vi "run.vi"(8 "error in (no error)":errorcluster, 11 "ScanModeTS090821Circular2D in":refnum<class "ImagingModeTS090821Circular2D.lvclass">) -> (0 "error out":errorcluster, 3 "ScanModeTS090821Circular2D out":refnum<class "ImagingModeTS090821Circular2D.lvclass">)   [LabVIEW 2010, in "ImagingModeTS090821Circular2D.lvclass"]
uses:
  ImagingModeTS090821Circular2D.lvclass
  common/classes/Image/Image/Image.lvclass
  GenericImagingMode/GenericImagingMode/GenericImagingMode.lvclass
  ImagingModeDL091001Scaffold/ImagingModeDL091001Scaffold/ImagingModeDL091001Scaffold.lvclass
  ImagingModeDL091001Scaffold/ImagingModeDL091001Scaffold_statechart.lvsc/Trigger.ctl
  ImagingModeDL091001Scaffold/ImagingModeDL091001Scaffold_statechart.lvsc
  bricks/enumerations/control_status.ctl
panel:
  in  "Tab Control":enum32{"User", "Debug", "About"}(tab)
  in  "save settings button":bool
  in  "load settings button":bool
  in  "number of cycles":i32=100
  in  "default settings":string(combo)
  in  "load image button":bool
  out "reference image":T1(plugin-control)
  in  "y amplitude":dbl[unit]=9.999999999999999e-06
  in  "x frequency":dbl=1.0
  in  "y frequency":dbl=1.0
  in  "phase shift":dbl
  in  "number of pixels per cycle":i32=250 min=0
  in  "x amplitude":dbl[unit]=9.999999999999999e-06
  in  "y center":dbl
  in  "x center":dbl
  in  "z center":dbl
  in  "rotation angle":dbl
  in  "type of trajectory":T2(radio)=enum."line (2-click)"
  in  "lines / frame":i32
  in  "spiral?":bool
  in  "dump factor":dbl=1.1
  in  "scanning frequency":dbl[unit]=5.0 min=0.0
  in  "pixel dwell time":dbl[unit]
  out "current frame":i32
  in  "Double":bool
  out "event loop error":errorcluster
  out "event handling loop counter":i32=10
  out "Type":i32(ring) items=["No Event"=0, "Click Event"=1, "Draw Event"=2, "Size Event"=4, "Scroll Event"=5, "Double Click Event"=8]
  out "Coordinates":i32[](array[numeric])
  in  "status":T3
  out "Tool":i32(ring) items=["None", "Selection Tool", "Point Tool", "Line Tool", "Rectangle Tool", "Oval Tool", "Polygon Tool", "ClosedFreehandTool", "Annulus Tool", "Rotated Rectangle Tool", "Zoom Tool", "Pan Tool", "Polyline Tool", "Freehand Tool"]
  out "finished?":bool
  out "x = y?":bool
  # "trajectory parameters"
  # "scan parameters"
  # "centering"
  # "spiral"
  # "ImagingModeTS090821Circular2D"
  # "Implemented by:\nTomasz Soltysinski, University Hospital Zurich, Switzerland"
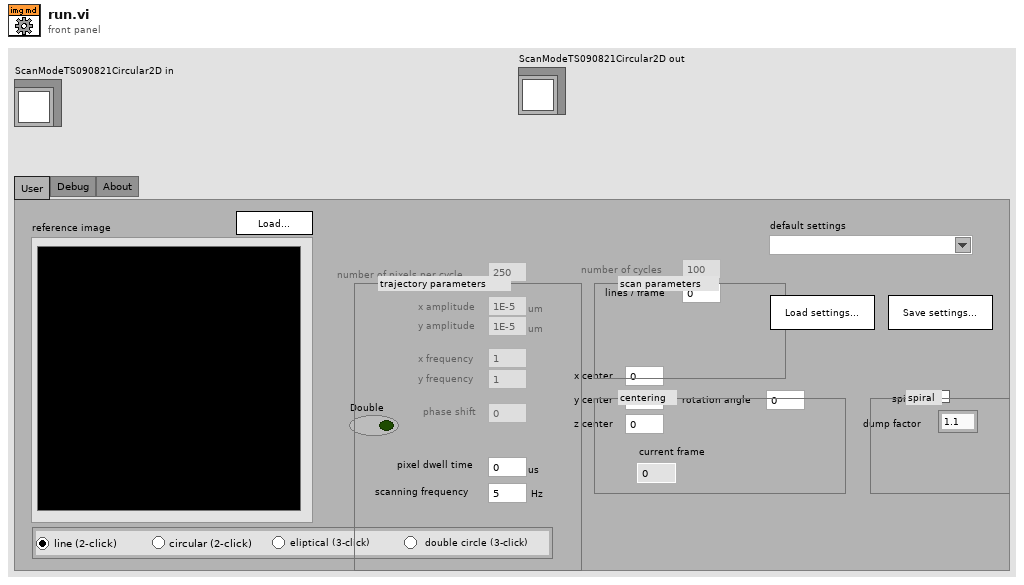
[diagram p1: front panel]
types:
  T1 = typedef "IMAQ Image.ctl" = refnum<image>
  T2 = enum32{"No Selection", "line (2-click)", "circular (2-click)", "eliptical (3-click)", "double circle (3-click)"}
  T3 = typedef "control_status.ctl" = enum16{"enabled", "disabled", "disabled & greyed out"}
  T4 = typedef "ImagingModeDL091001Scaffold_statechart.lvsc/Trigger.ctl" = enum16{"NULL", "initialise", "terminate", "start sweep", "stop sweep", "update", "proceed", "draw overlay"}
  T5 = enum8{"Enabled", "Disabled", "Disabled and Grayed Out"}
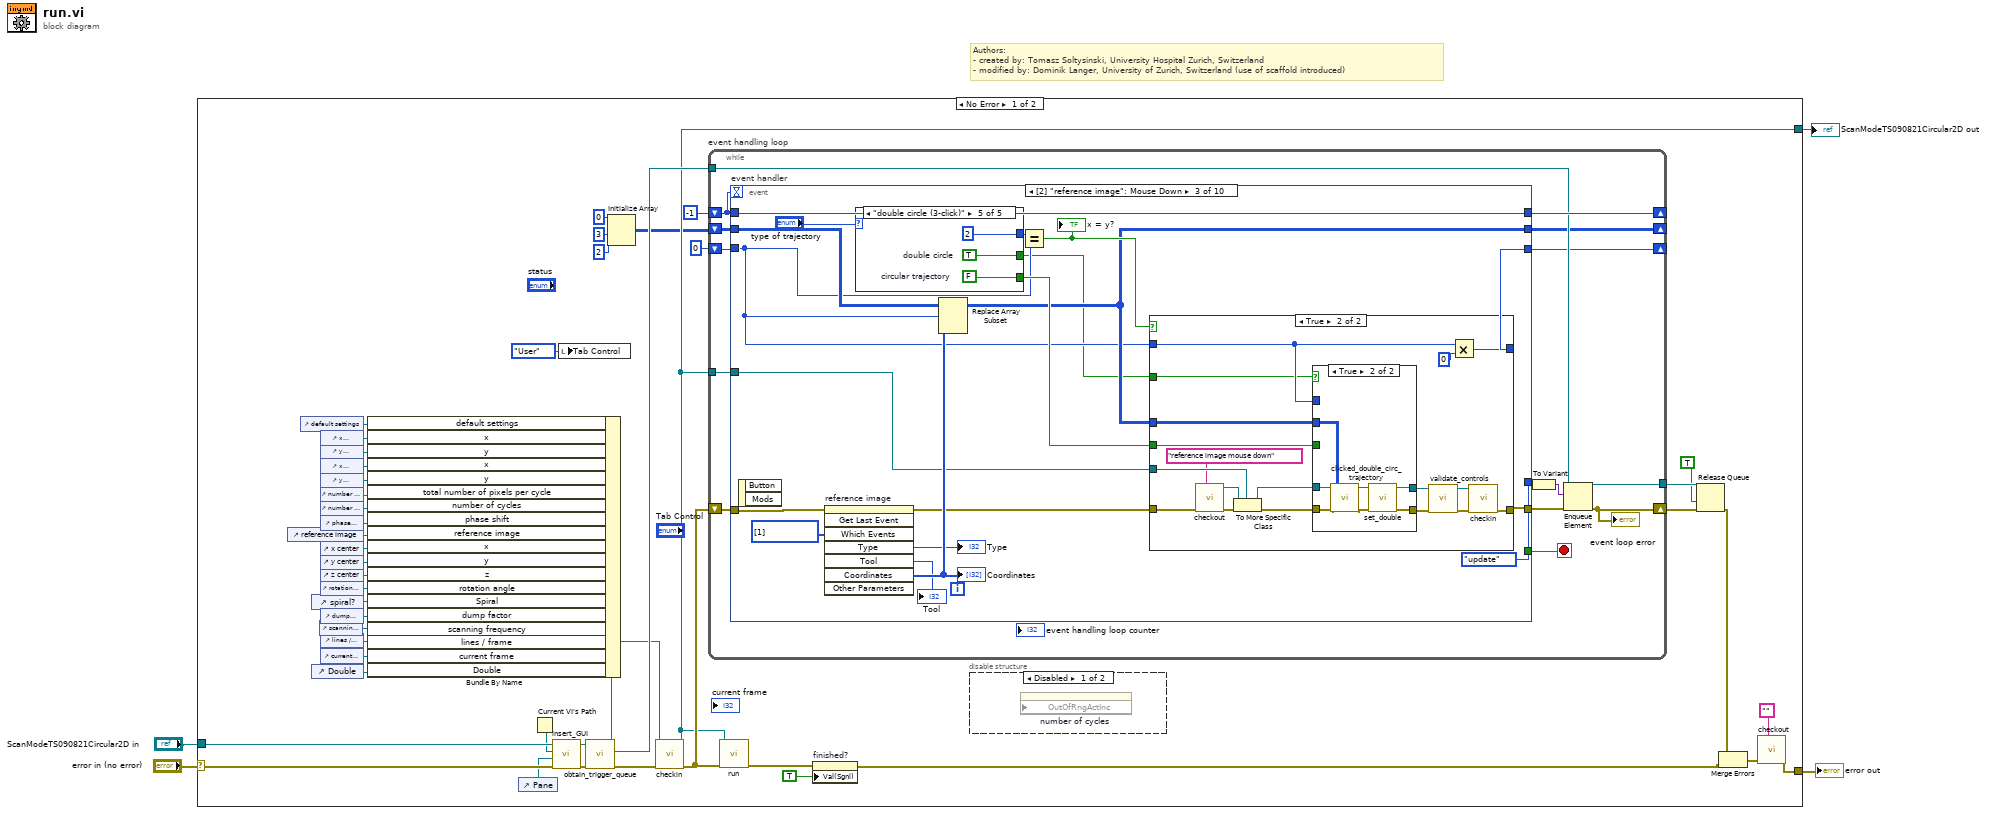
[diagram p0: block diagram]
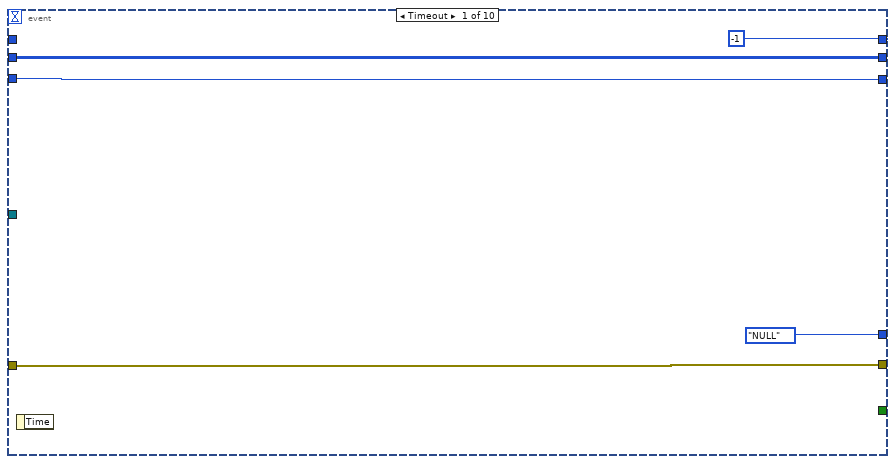
[diagram p3: hidden frame]
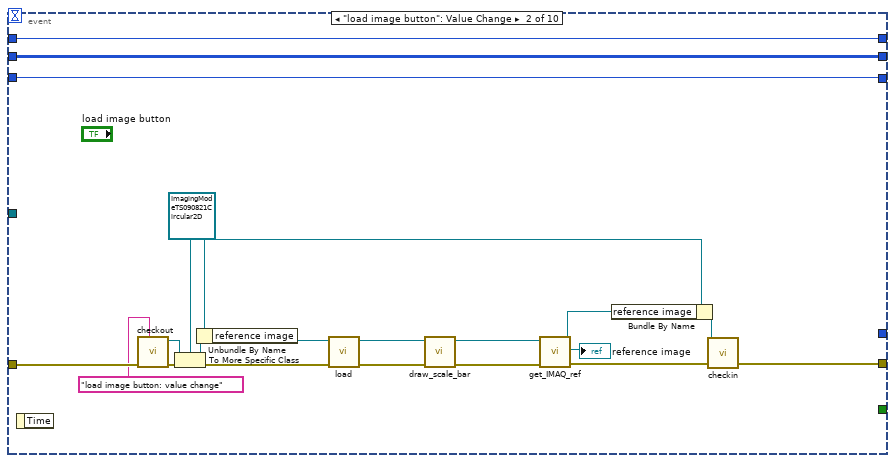
[diagram p4: hidden frame]
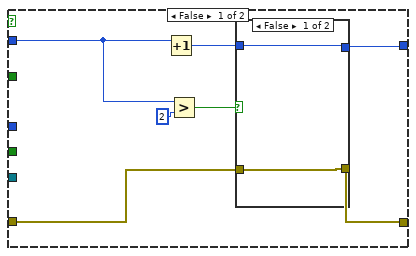
[diagram p5: hidden frame]
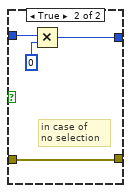
[diagram p6: hidden frame]
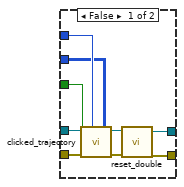
[diagram p7: hidden frame]
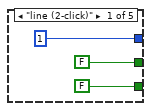
[diagram p8: hidden frame]
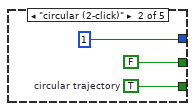
[diagram p9: hidden frame]
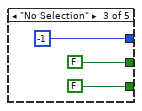
[diagram p10: hidden frame]
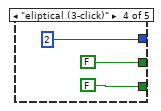
[diagram p11: hidden frame]
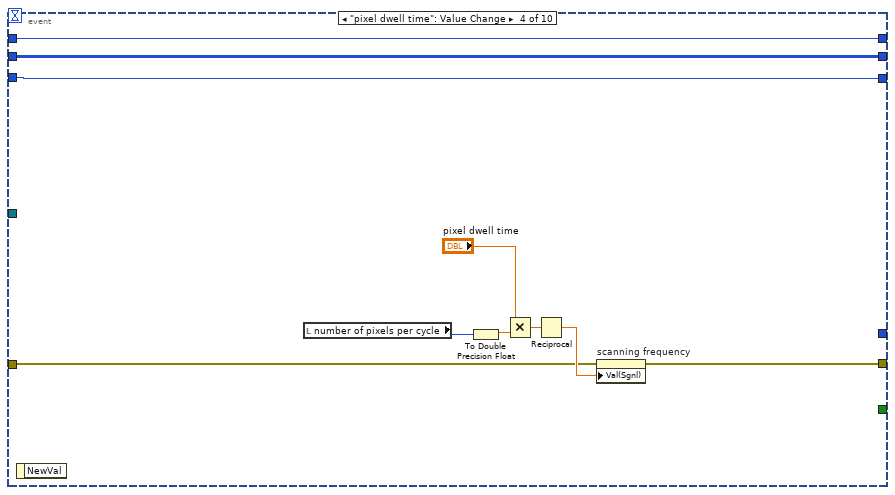
[diagram p12: hidden frame]
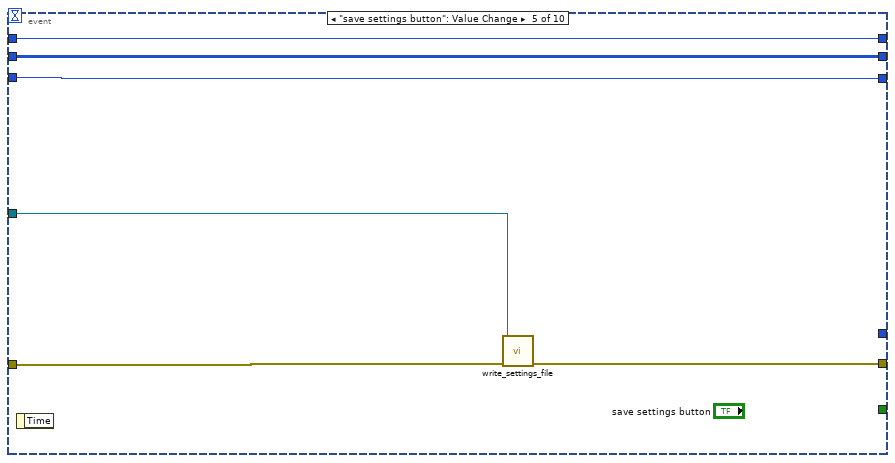
[diagram p13: hidden frame]
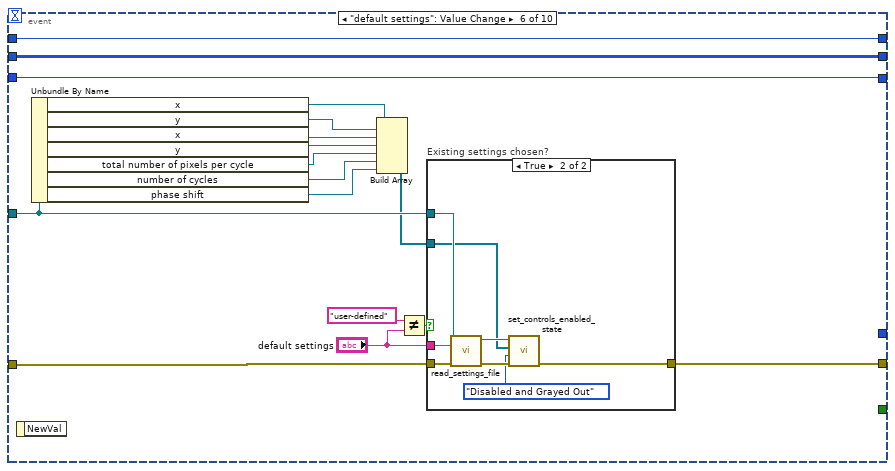
[diagram p14: hidden frame]
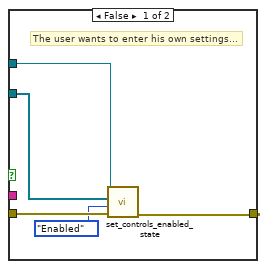
[diagram p15: hidden frame]
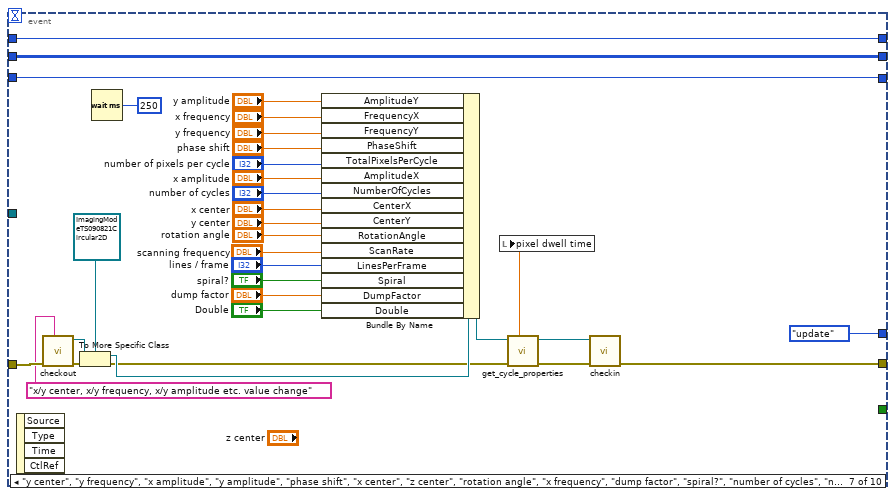
[diagram p16: hidden frame]
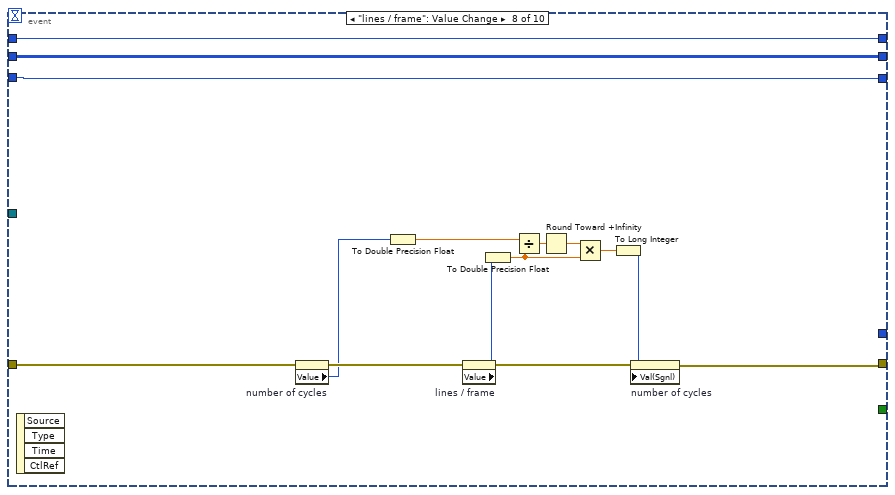
[diagram p17: hidden frame]
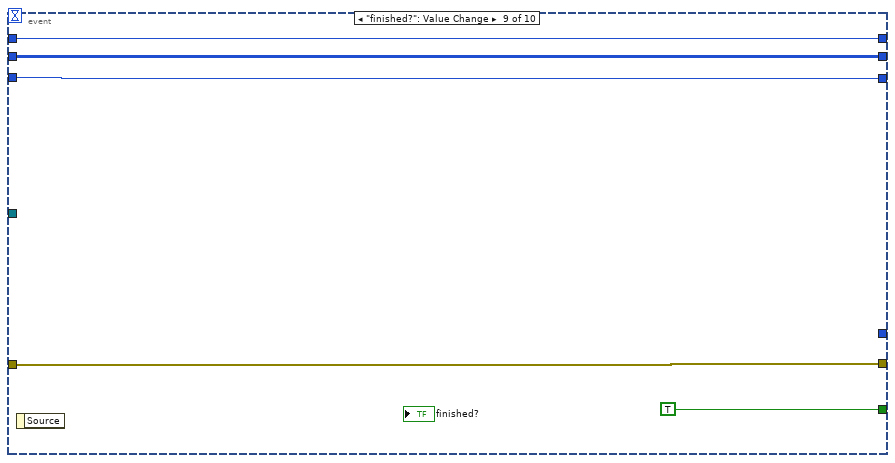
[diagram p18: hidden frame]
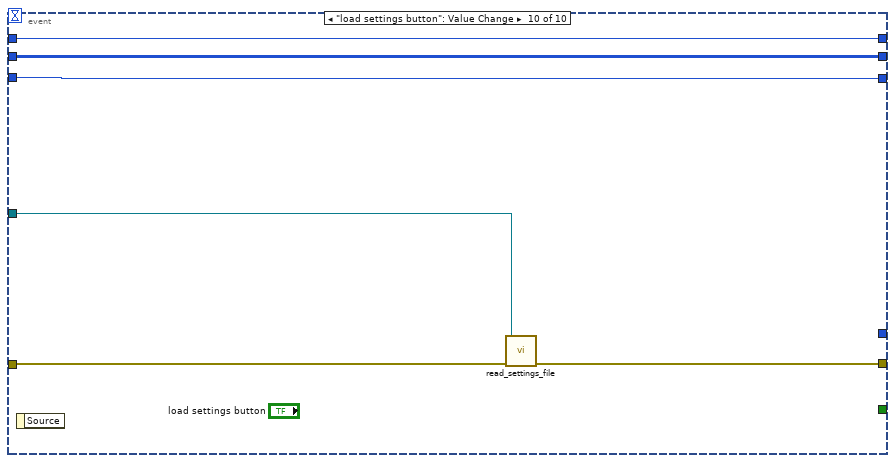
[diagram p19: hidden frame]
diagram:
  # "Authors: \n- created by: Tomasz Soltysinski, University Hospital Zurich, Switzerland\n- modified by: Dominik Langer, University of Zurich, Switzerland (use of scaffold introduced)"
  n1 = case shown="No Error" "error in (no error)" {
    selector: "error in (no error)" -> [w10 w279]
    tunnel: [w14 w279] -> w4
    tunnel: [w40 w278] -> w1
    tunnel: "ScanModeTS090821Circular2D in" -> [w9 w278]
    frame No Error {
      n2 = control-ref of="reference image"() -> (w26:refnum<vi>)
      n3 = control-ref of="default settings"() -> (w28:refnum<vi>)
      n4 = control-ref of="spiral?"() -> (w25:refnum<vi>)
      n5 = control-ref of="Double"() -> (w7:refnum<vi>)
      n6 = control-ref of="scanning frequency"() -> (w20:refnum<vi>)
      n7 = control-ref of="x amplitude"() -> (w35:refnum<vi>)
      n8 = control-ref of="y amplitude"() -> (w34:refnum<vi>)
      n9 = control-ref of="x frequency"() -> (w33:refnum<vi>)
      n10 = control-ref of="y frequency"() -> (w32:refnum<vi>)
      n11 = control-ref of="number of pixels per cycle"() -> (w31:refnum<vi>)
      n12 = control-ref of="number of cycles"() -> (w30:refnum<vi>)
      n13 = control-ref of="phase shift"() -> (w29:refnum<vi>)
      n14 = control-ref of="x center"() -> (w24:refnum<vi>)
      n15 = control-ref of="y center"() -> (w23:refnum<vi>)
      n16 = control-ref of="z center"() -> (w22:refnum<vi>)
      n17 = control-ref of="rotation angle"() -> (w27:refnum<vi>)
      n18 = control-ref of="dump factor"() -> (w21:refnum<vi>)
      n19 = control-ref of="lines / frame"() -> (w19:refnum<vi>)
      n20 = control-ref of="current frame"() -> (w18:refnum<vi>)
      n21 = control-ref of="Pane"() -> (w5:refnum<vi>)
      n22 = Current VI's Path() -> (path=w8:path)
      n23 = call-dynamic "insert_GUI.vi"("error in (no error)"=w10, "Pane"=w5, "VI path"=w8, "GenericComponent in"=w9) -> ("error out"=w12:errorcluster, "GenericComponent out"=w11:refnum<class "ImagingModeTS090821Circular2D.lvclass">)  [unwired: 6 in]
      n24 = local write "Tab Control"(enum32{"User", "Debug", "About"}."User" ("Tab Control")) -> ()
      n25 = call-dynamic "obtain_trigger_queue.vi"("error in (no error)"=w12, "GenericPlugin in"=w11) -> ("error out"=w43:errorcluster, "trigger queue"=w41:refnum<queue>, "GenericPlugin out"=w17:refnum<class "ImagingModeTS090821Circular2D.lvclass">)  [unwired: 7 in]
      n26 = Bundle By Name(cluster=w17, "default settings"=w28, "x"=w35, "y"=w34, "x"=w33, "y"=w32, "total number of pixels per cycle"=w31, "number of cycles"=w30, "phase shift"=w29, "reference image"=w26, "x"=w24, "y"=w23, "z"=w22, "rotation angle"=w27, "Spiral"=w25, "dump factor"=w21, "scanning frequency"=w20, "lines / frame"=w19, "current frame"=w18, "Double"=w7) -> (w16:refnum<class "ImagingModeTS090821Circular2D.lvclass">)
      n27 = Initialize Array(0, 3 ("dimension size"), 2 ("dimension size")) -> (w36:i32[][])
      n28 = call "checkin.vi"("error in (no error)"=w43, "GenericScanMode in"=w16) -> ("error out"=w42:errorcluster, "GenericScanMode out"=w40:refnum<class "ImagingModeTS090821Circular2D.lvclass">)  [unwired: 8 in]
      n29 = while "event handling loop" {
        shift-right: [w66] -> _
        shift-left: -1 -> [w67]
        shift-right: [w59] -> w51
        shift-left: w42 -> [w65]
        tunnel: w41 -> [w63]
        tunnel: [w61] -> w50
        tunnel: w40 -> [w60]
        shift-right: [w58] -> _
        shift-left: w36 -> [w57]
        shift-right: [w55] -> _
        shift-left: 0 -> [w56]
        stop <- w64 stop-if-true
        n30 = event "event handler" shown="[2] \"reference image\": Mouse Down" {
          selector: _ -> [_ _ _ _ _ _ _ _ _ _]
          dyn-events: _ -> [_ _ _ _ _ _ _ _ _ _]
          timeout: w67 -> [_ _ _ _ _ _ _ _ _ _]
          tunnel: [-1 w92 w111 w183 w189 w206 w251 w266 w271 w277] -> w66
          tunnel: w67 -> [_ w92 w111 w183 w189 w206 w251 w266 w271 w277]
          tunnel: w65 -> [w71 w87 w103 w176 w188 w205 w239 w262 w270 w275]
          tunnel: [w71 w79 w106 w180 w187 w204 w238 w252 w270 w274] -> w62
          tunnel: [_ _ _ _ _ _ _ _ TRUE _] -> w64
          tunnel: w60 -> [_ _ w96 _ w186 w191 _ _ _ w276]
          tunnel: [Trigger."NULL" ("Trigger") _ Trigger."update" ("Trigger") _ _ _ Trigger."update" ("Trigger") _ _ _] -> w54
          tunnel: [w70 w81 w107 w182 w185 w200 w234 w265 w268 w273] -> w58
          tunnel: w57 -> [w70 w81 w102 w182 w185 w200 w234 w265 w268 w273]
          tunnel: w56 -> [w69 w80 w100 w181 w184 w199 w233 w264 w267 w272]
          tunnel: [w69 w80 w104 w181 w184 w199 w233 w264 w267 w272] -> w55
          event Timeout {
            n31 = event-data() -> ()  [unwired: 2 out]
          }
          event "load image button": Value Change {
            n32 = event-data() -> ()  [unwired: 2 out]
            n33 = call "checkout.vi"("locked by?"="load image button: value change", "error in (no error)"=w87) -> ("error out"=w91:errorcluster, "GenericScanMode out"=w90:refnum<class "GenericImagingMode.lvclass">)  [unwired: 8 in]
            n34 = To More Specific Class(target class=refnum<class "ImagingModeTS090821Circular2D.lvclass"> refnum ("ScanModeTS090821Circular2D.lvclass"), reference=w90, error in=w91) -> (specific class reference=w82:refnum<class "ImagingModeTS090821Circular2D.lvclass">, error out=w86:errorcluster)
            n35 = Unbundle By Name(w82) -> ("reference image"=w88:refnum<class "Image.lvclass">)
            n36 = call-dynamic "load.vi"("error in (no error)"=w86, "Image in"=w88) -> ("error out"=w76:errorcluster, "Image out"=w74:refnum<class "Image.lvclass">)  [unwired: 6 in, 2 out]
            n37 = call "draw_scale_bar.vi"("error in (no error)"=w76, "Image in"=w74) -> ("error out"=w75:errorcluster, "Image out"=w73:refnum<class "Image.lvclass">)  [unwired: 8 in]
            n38 = call-dynamic "get_IMAQ_ref.vi"("error in (no error)"=w75, "Image.lvclass in"=w73) -> ("error out"=w78:errorcluster, "Image"=→"reference image":T1, "Image.lvclass out"=w85:refnum<class "Image.lvclass">)  [unwired: 5 in, 2 out]
            n39 = Bundle By Name(cluster=w82, "reference image"=w85) -> (w77:refnum<class "ImagingModeTS090821Circular2D.lvclass">)
            n40 = call "checkin.vi"("error in (no error)"=w78, "GenericScanMode in"=w77) -> ("error out"=w79:errorcluster)  [unwired: 8 in, 1 out]
          }
          event "reference image": Mouse Down {
            w97 = i32[] [1] items=["No  event", "Click event", "Draw event", "Move event", "Size event", "Scroll event", "Activate event", "Close event", "Double click event"] ("Events list (all)")
            n41 = event-data() -> ()  [unwired: 3 out]
            n42 = invoke on="reference image" class="ImageControl" method="Get Last Event"(error in=w103, "Which Events"=w97) -> (error out=w95:errorcluster, "Type"=→"Type":i32, "Tool"=→"Tool":i32, "Coordinates"=w101:i32[])  [unwired: 6 in, 4 out]
            "Coordinates" <- w101
            n43 = case shown="\"double circle (3-click)\"" "type of trajectory" {
              tunnel: [1 1 -1 2 2] -> w110
              tunnel: [FALSE w163 FALSE ("circular trajectory") FALSE ("circular trajectory") w172] -> w109
              tunnel: [FALSE ("double circle") FALSE ("double circle") FALSE ("double circle") FALSE ("double circle") w171] -> w94
              frame "line (2-click)" {
              }
              frame "circular (2-click)" {
                w163 = TRUE  # circular trajectory
              }
              frame "No Selection" {
              }
              frame "eliptical (3-click)" {
              }
              frame "double circle (3-click)" {
                w171 = TRUE  # double circle
                w172 = FALSE  # circular trajectory
              }
            }
            n44 = Replace Array Subset(array=w102, new element=w101, index (row)=w100) -> (w107:i32[][])  [unwired: 1 in]
            n45 = Equal?(x=w110, y=w100) -> (x = y?=w108:bool)
            "x = y?" <- w108
            n46 = case shown="True" w108 {
              tunnel: [w117 w142] -> w104
              tunnel: w100 -> [w113 w140]
              tunnel: w107 -> [_ w139]
              tunnel: w96 -> [_ w131]
              tunnel: w95 -> [w115 w135]
              tunnel: [w114 w129] -> w106
              tunnel: w109 -> [_ w138]
              tunnel: w94 -> [_ w125]
              frame False {
                n47 = Increment(x=w113) -> (x+1=w118:i32)
                n48 = Greater?(x=w113, y=2) -> (0:w116:bool)
                n49 = case shown="False" w116 {
                  tunnel: w118 -> [w120 w123]
                  tunnel: [w120 w122] -> w117
                  tunnel: w115 -> [w119 w121]
                  tunnel: [w119 w121] -> w114
                  frame False {
                  }
                  frame True {
                    # "in case of\nno selection"
                    n50 = Multiply(x=w123, y=0 ("x")) -> (x*y=w122:i32)
                  }
                }
              }
              frame True {
                n51 = call "checkout.vi"("locked by?"="reference image mouse down", "error in (no error)"=w135) -> ("error out"=w134:errorcluster, "GenericScanMode out"=w132:refnum<class "GenericImagingMode.lvclass">)  [unwired: 8 in]
                n52 = To More Specific Class(target class=w131, reference=w132, error in=w134) -> (specific class reference=w127:refnum<class "ImagingModeTS090821Circular2D.lvclass">, error out=w133:errorcluster)
                n53 = case shown="True" w125 {
                  tunnel: w140 -> [w151 _]
                  tunnel: w139 -> [w150 w157]
                  tunnel: w138 -> [w149 _]
                  tunnel: [w143 w154] -> w137
                  tunnel: [w145 w152] -> w136
                  tunnel: w133 -> [w148 w158]
                  tunnel: w127 -> [w147 w156]
                  frame False {
                    n54 = call-dynamic "clicked_trajectory.vi"("ScanModeTS090821Circular2D in"=w147, "clicked points"=w150, "Numeric"=w151, "circular trajectory"=w149, "error in (no error)"=w148) -> ("ScanModeTS090821Circular2D out"=w146:refnum<class "ImagingModeTS090821Circular2D.lvclass">, "error out"=w144:errorcluster)  [unwired: 21 in]
                    n55 = call-dynamic "reset_double.vi"("error in (no error)"=w144, "ImagingModeTS090821Circular2D in"=w146) -> ("error out"=w143:errorcluster, "ImagingModeTS090821Circular2D out"=w145:refnum<class "ImagingModeTS090821Circular2D.lvclass">)  [unwired: 8 in]
                  }
                  frame True {
                    n56 = call-dynamic "clicked_double_circ_trajectory.vi"("ScanModeTS090821Circular2D in"=w156, "clicked points"=w157, "error in (no error)"=w158) -> ("ScanModeTS090821Circular2D out"=w153:refnum<class "ImagingModeTS090821Circular2D.lvclass">, "error out"=w155:errorcluster)  [unwired: 23 in]
                    n57 = call-dynamic "set_double.vi"("error in (no error)"=w155, "ImagingModeTS090821Circular2D in"=w153) -> ("error out"=w154:errorcluster, "ImagingModeTS090821Circular2D out"=w152:refnum<class "ImagingModeTS090821Circular2D.lvclass">)  [unwired: 8 in]
                  }
                }
                n58 = call-dynamic "validate_controls.vi"("error in (no error)"=w137, "ScanModeTS090821Circular2D in"=w136) -> ("error out"=w130:errorcluster, "ScanModeTS090821Circular2D out"=w128:refnum<class "ImagingModeTS090821Circular2D.lvclass">)  [unwired: 8 in]
                n59 = Multiply(x=w140, y=0) -> (x*y=w142:i32)
                n60 = call "checkin.vi"("error in (no error)"=w130, "GenericScanMode in"=w128) -> ("error out"=w129:errorcluster)  [unwired: 8 in, 1 out]
              }
            }
          }
          event "pixel dwell time": Value Change {
            n61 = event-data() -> ()  [unwired: 2 out]
            n62 = local read "number of pixels per cycle"() -> (w175:i32)
            n63 = To Double Precision Float(number=w175) -> (double precision float=w179:dbl)
            n64 = Multiply(x="pixel dwell time", y=w179) -> (x*y=w178:dbl[unit])
            n65 = Reciprocal(x=w178) -> (1/x=w177:dbl[unit])
            n66 = property on="scanning frequency" class="DigNum (strict)"(error in=w176, "Val(Sgnl)"=w177) -> (error out=w180:errorcluster)  [unwired: 1 in, 1 out]
          }
          event "save settings button": Value Change {
            n67 = event-data() -> ()  [unwired: 2 out]
            n68 = call-dynamic "write_settings_file.vi"("error in (no error)"=w188, "GenericPlugin in"=w186) -> ("error out"=w187:errorcluster)  [unwired: 6 in, 3 out]
          }
          event "default settings": Value Change {
            n69 = event-data() -> ()  [unwired: 2 out]
            n70 = Unbundle By Name(w191) -> ("x"=w198:refnum<vi>, "y"=w197:refnum<vi>, "x"=w196:refnum<vi>, "y"=w195:refnum<vi>, "total number of pixels per cycle"=w194:refnum<vi>, "number of cycles"=w193:refnum<vi>, "phase shift"=w192:refnum<vi>)
            n71 = Build Array(w198, w197, w196, w195, w194, w193, w192) -> (w190:refnum<vi>[])
            n72 = Not Equal?(x="user-defined", y="default settings") -> (x != y?=w202:bool)
            n73 = case "Existing settings chosen?" shown="True" w202 {
              tunnel: w191 -> [w210 w215]
              tunnel: w205 -> [w211 w217]
              tunnel: [w209 w219] -> w204
              tunnel: "default settings" -> [_ w214]
              tunnel: w190 -> [w207 w212]
              frame False {
                # "The user wants to enter his own settings..."
                n74 = call-dynamic "set_controls_enabled_state.vi"("error in (no error)"=w211, "status"=T5."Enabled", "control references"=w207, "GenericPlugin in"=w210) -> ("error out"=w209:errorcluster)  [unwired: 6 in, 1 out]
              }
              frame True {
                n75 = call-dynamic "read_settings_file.vi"("error in (no error)"=w217, "settings name"=w214, "ScanModeTS090821Circular2D in"=w215) -> ("error out"=w218:errorcluster, "ScanModeTS090821Circular2D out"=w216:refnum<class "ImagingModeTS090821Circular2D.lvclass">)  [unwired: 6 in, 1 out]
                n76 = call-dynamic "set_controls_enabled_state.vi"("error in (no error)"=w218, "status"=T5."Disabled and Grayed Out", "control references"=w212, "GenericPlugin in"=w216) -> ("error out"=w219:errorcluster)  [unwired: 6 in, 1 out]
              }
            }
          }
          event "y center", "y frequency", "x amplitude", "y amplitude", "phase shift", "x center", "z center", "rotation angle", "x frequency", "dump factor", "spiral?", "number of cycles", "number of pixels per cycle", "scanning frequency": Value Change {
            n77 = event-data() -> ()  [unwired: 5 out]
            n78 = call "checkout.vi"("locked by?"="x/y center, x/y frequency, x/y amplitude etc. value change", "error in (no error)"=w239) -> ("error out"=w250:errorcluster, "GenericScanMode out"=w249:refnum<class "GenericImagingMode.lvclass">)  [unwired: 8 in]
            n79 = To More Specific Class(target class=refnum<class "ImagingModeTS090821Circular2D.lvclass"> refnum ("ScanModeTS090821Circular2D.lvclass"), reference=w249, error in=w250) -> (specific class reference=w246:refnum<class "ImagingModeTS090821Circular2D.lvclass">, error out=w227:errorcluster)
            n80 = Wait (ms)(milliseconds to wait=u32 250) -> ()  [unwired: 1 out]
            n81 = Bundle By Name(cluster=w246, "AmplitudeY"="y amplitude", "FrequencyX"="x frequency", "FrequencyY"="y frequency", "PhaseShift"="phase shift", "TotalPixelsPerCycle"="number of pixels per cycle", "AmplitudeX"="x amplitude", "NumberOfCycles"="number of cycles", "CenterX"="x center", "CenterY"="y center", "RotationAngle"="rotation angle", "ScanRate"="scanning frequency", "LinesPerFrame"="lines / frame", "Spiral"="spiral?", "DumpFactor"="dump factor", "Double"="Double") -> (w225:refnum<class "ImagingModeTS090821Circular2D.lvclass">)
            n82 = call-dynamic "get_cycle_properties.vi"("error in (no error)"=w227, "ScanModeTS090821Circular2D in"=w225) -> ("error out"=w226:errorcluster, "ScanModeTS090821Circular2D out"=w224:refnum<class "ImagingModeTS090821Circular2D.lvclass">, "pixel dwell time"=w223:dbl[unit])  [unwired: 3 in, 4 out]
            n83 = local write "pixel dwell time"(w223) -> ()
            n84 = call "checkin.vi"("error in (no error)"=w226, "GenericScanMode in"=w224) -> ("error out"=w238:errorcluster)  [unwired: 8 in, 1 out]
          }
          event "lines / frame": Value Change {
            n85 = event-data() -> ()  [unwired: 5 out]
            n86 = property on="number of cycles" class="DigNum (strict)"(error in=w262) -> (error out=w261:errorcluster, "Value"=w260:i32)  [unwired: 1 in, 1 out]
            n87 = To Double Precision Float(number=w260) -> (double precision float=w259:dbl)
            n88 = property on="lines / frame" class="DigNum (strict)"(error in=w261) -> (error out=w256:errorcluster, "Value"=w263:i32)  [unwired: 1 in, 1 out]
            n89 = To Double Precision Float(number=w263) -> (double precision float=w254:dbl)
            n90 = Divide(x=w259, y=w254) -> (x/y=w258:dbl)
            n91 = Round Toward +Infinity(x=w258) -> (ceil(x): smallest int >= x=w253:dbl)
            n92 = Multiply(x=w253, y=w254) -> (x*y=w255:dbl)
            n93 = To Long Integer(number=w255) -> (32bit integer=w257:i32)
            n94 = property on="number of cycles" class="DigNum (strict)"(error in=w256, "Val(Sgnl)"=w257) -> (error out=w252:errorcluster)  [unwired: 1 in, 1 out]
          }
          event "finished?": Value Change {
            n95 = event-data() -> ()  [unwired: 2 out]
          }
          event "load settings button": Value Change {
            n96 = event-data() -> ()  [unwired: 2 out]
            n97 = call-dynamic "read_settings_file.vi"("error in (no error)"=w275, "ScanModeTS090821Circular2D in"=w276) -> ("error out"=w274:errorcluster)  [unwired: 7 in, 2 out]
          }
        }
        n98 = To Variant(anything=w54) -> (Variant=w53:variant)
        n99 = Enqueue Element(queue=w63, element=w53, error in (no error)=w62) -> (queue out=w61:refnum<queue>, error out=w59:errorcluster)  [unwired: 2 out]
        "event loop error" <- w59
      }
      n100 = call-parent "run.vi"("error in (no error)"=w42, "ScanModeDL091001Scaffold in"=w40) -> ("error out"=w45:errorcluster)  [unwired: 8 in, 1 out]
      n101 = property on="finished?" class="Bool (strict)"(error in=w45, "Val(Sgnl)"=TRUE) -> (error out=w13:errorcluster)  [unwired: 1 in, 1 out]
      n102 = disable-structure shown="Disabled" {
        frame Disabled {
          n103 = property on="number of cycles" class="DigNum (strict)" props=["OutOfRngActInc"]() -> ()  [unwired: 3 in, 2 out]
        }
        frame Enabled {
        }
      }
      n104 = Release Queue(queue=w50, force destroy? (F)=TRUE, error in (no error)=w51) -> (error out=w48:errorcluster)  [unwired: 2 out]
      n105 = Merge Errors(w48, w13) -> (w15:errorcluster)
      n106 = call "checkout.vi"("locked by?"="", "error in (no error)"=w15) -> ("error out"=w14:errorcluster)  [unwired: 8 in, 1 out]
    }
    frame Error {
    }
  }
  "error out" <- w4
  "ScanModeTS090821Circular2D out" <- w1
